vi "flatten range.vi"(9 "output low":dbl, 10 "output high":dbl, 11 "ID":string) -> (3 "wrapped data":string)   [LabVIEW 2013, in "PID Loop.lvclass"]
uses:
  PID Loop.lvclass
  <vilib>/NI/Configuration Framework/serializable configuration/NISE_CEF_serializable configuration.lvclass
  String Parameters.ctl
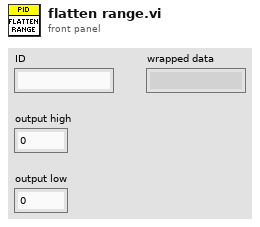
[diagram p1: front panel]
types:
  T1 = typedef "PID Loop.lvclass/String Parameters.ctl" = enum16{"Setpoint", "Process Variable", "Output", "Proportional Gain", "Integral Time", "Derivative Time", "Range High", "Range Low"}
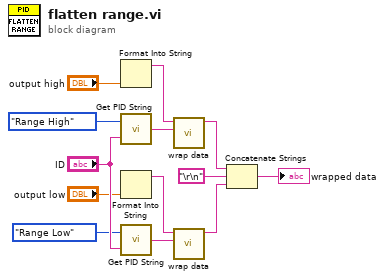
[diagram p0: block diagram]
diagram:
  n1 = Format Into String("output high") -> (resulting string=w6:string)  [unwired: 3 in, 1 out]
  n2 = call "Get PID String.vi"("PID Loop ID"="ID", "PID Parameter"=String_Parameters."Range High") -> ("Parameter String"=w7:string)
  n3 = Format Into String("output low") -> (resulting string=w4:string)  [unwired: 3 in, 1 out]
  n4 = call "Get PID String.vi"("PID Loop ID"="ID", "PID Parameter"=String_Parameters."Range Low") -> ("Parameter String"=w2:string)
  n5 = call <vilib>:"wrap data.vi"("identifier"=w7, "data to wrap"=w6) -> ("wrapped data"=w11:string)  [unwired: 9 in]
  n6 = call <vilib>:"wrap data.vi"("identifier"=w2, "data to wrap"=w4) -> ("wrapped data"=w12:string)  [unwired: 9 in]
  n7 = Concatenate Strings(w11, "\r\n", w12) -> (→"wrapped data":string)
